vi "Get Position.vi"(6 "Counter Time":i32, 8 "error in (no error)":errorcluster, 9 "Piezo State":T2, 10 "notifier out":refnum<notifier>, 11 "Hardware Resources In":T1={"Piezo Serial Number"=41848555, "MG17Piezo"=refnum, "Setpoint (um)"=0.0}) -> (0 "error out":errorcluster, 3 "Hardware Resources Out":T1={"Piezo Serial Number"=41848555, "MG17Piezo"=refnum, "Setpoint (um)"=0.0})   [LabVIEW 2013, in "Piezo.lvlib"]
uses:
  Piezo.lvlib
  Piezo State.ctl
  Hardware Configuration.ctl
  Piezo display.ctl
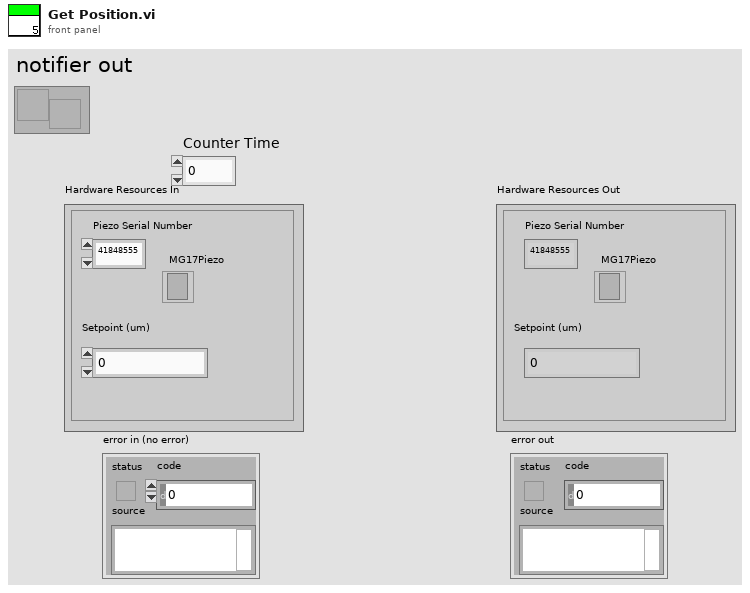
[diagram p1: front panel]
types:
  T1 = typedef "Piezo.lvlib/Hardware Configuration.ctl" = cluster{"Piezo Serial Number":i32, "MG17Piezo":refnum<k7>, "Setpoint (um)":sgl}
  T2 = typedef "Piezo.lvlib/Piezo State.ctl" = enum16{"Idle", "Acquiring"}
  T3 = typedef "Piezo.lvlib/Piezo display.ctl" = cluster{"PiezoPosition":sgl, "Counter Time":i32}
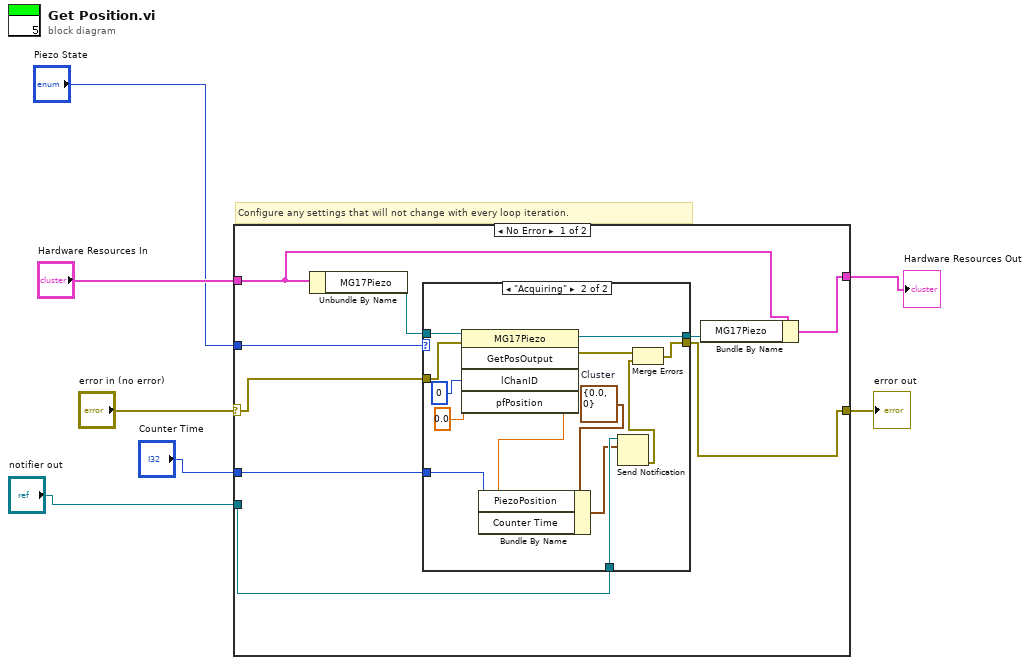
[diagram p0: block diagram]
diagram:
  # "Configure any settings that will not change with every loop iteration."
  n1 = case shown="No Error" "error in (no error)" {
    selector: "error in (no error)" -> [w12 w33]
    tunnel: [w9 w33] -> w6
    tunnel: [w14 w32] -> w4
    tunnel: "Hardware Resources In" -> [w15 w32]
    tunnel: "Piezo State" -> [w11 _]
    tunnel: "notifier out" -> [w10 _]
    tunnel: "Counter Time" -> [w8 _]
    frame No Error {
      n2 = Unbundle By Name(w15) -> ("MG17Piezo"=w16:refnum<k7>)
      n3 = case shown="\"Acquiring\"" w11 {
        tunnel: w16 -> [w18 w31]
        tunnel: [w18 w30] -> w13
        tunnel: [w17 w24] -> w9
        tunnel: w12 -> [w17 w29]
        tunnel: w10 -> [_ w27]
        tunnel: w8 -> [_ w19]
        frame "Idle", Default {
        }
        frame "Acquiring" {
          w20 = T3 {"PiezoPosition"=0.0, "Counter Time"=0}  # Cluster
          n4 = invoke class="MG17Piezo" method="GetPosOutput"(reference=w31, error in=w29, "lChanID"=0, "pfPosition"=sgl 0.0) -> (reference out=w30:refnum<k7>, error out=w22:errorcluster, "pfPosition"=w26:sgl)  [unwired: 1 in, 2 out]
          n5 = Bundle By Name(cluster=w20, "PiezoPosition"=w26, "Counter Time"=w19) -> (w21:T3)
          n6 = Send Notification(notification=w21, notifier=w27) -> (error out=w23:errorcluster)  [unwired: 1 in, 1 out]
          n7 = Merge Errors(w22, w23) -> (w24:errorcluster)
        }
      }
      n8 = Bundle By Name(cluster=w15, "MG17Piezo"=w13) -> (w14:T1)
    }
    frame Error {
    }
  }
  "error out" <- w6
  "Hardware Resources Out" <- w4
